vi "Disable and Gray.vi"(7 "Disabled":T1(ring)=enum."Disabled and Grayed Out", 8 "error in (no error)":errorcluster, 11 "Refnum VI":refnum<vi>) -> (0 "error out":errorcluster)   [LabVIEW 2020]
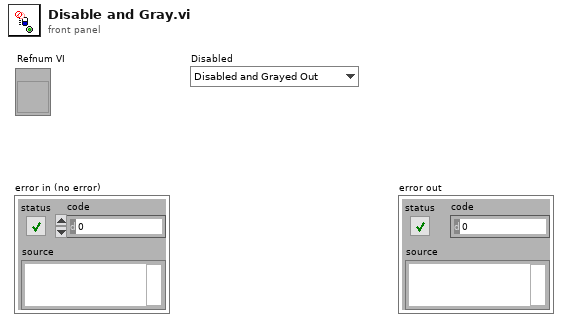
[diagram p1: front panel]
types:
  T1 = enum8{"Enabled", "Disabled", "Disabled and Grayed Out"}
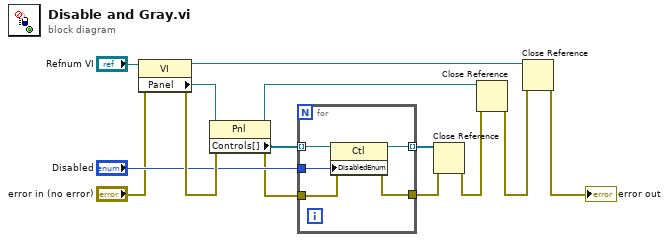
[diagram p0: block diagram]
diagram:
  n1 = property class="VI"(reference="Refnum VI", error in="error in (no error)") -> (reference out=w4:refnum<vi>, error out=w12:errorcluster, "Panel"=w13:refnum<vi>)
  n2 = property class="Pnl"(reference=w13, error in=w12) -> (reference out=w3:refnum<vi>, error out=w9:errorcluster, "Controls[]"=w11:refnum<vi>[])
  n3 = for {
    tunnel: w11 -> [w19] mode=indexing
    tunnel: "Disabled" -> [w18]
    tunnel: w9 -> [w17]
    tunnel: [w16] -> w8
    tunnel: [w15] -> w7 mode=indexing
    n4 = property class="Ctl"(reference=w19, error in=w17, "DisabledEnum"=w18) -> (reference out=w15:refnum<vi>, error out=w16:errorcluster)
  }
  n5 = Close Reference(reference=w7, error in (no error)=w8) -> (error out=w6:errorcluster)
  n6 = Close Reference(reference=w3, error in (no error)=w6) -> (error out=w5:errorcluster)
  n7 = Close Reference(reference=w4, error in (no error)=w5) -> (error out=→"error out":errorcluster)
